vi "Emulate Licor output GV.vi"() -> ()   [LabVIEW 2017, in "Licor-Steuerung.lvlib"]
uses:
  Licor-Steuerung.lvlib
  LicorLI7000/conventions/output line.ctl
  LicorLI7000/LicorLI7000.lvlib
panel:
  in  "Emulator Daten":T1[](array[typedef]) {"time (global)" format="%<%H:%M:%S\n%d/%m/%Y>T"}
  in  "Emulator an?":bool
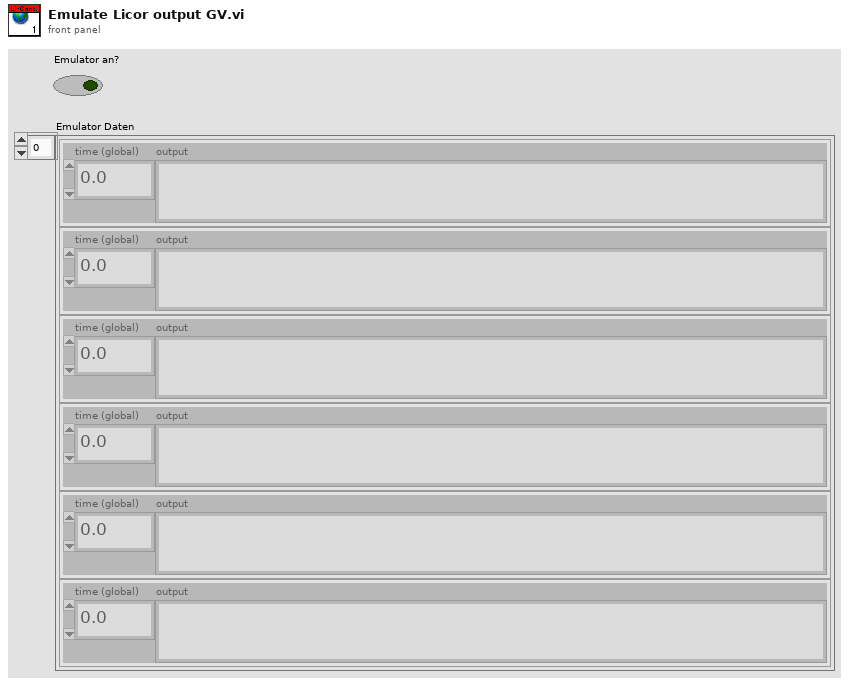
[diagram p1: front panel]
types:
  T1 = typedef "LicorLI7000.lvlib/output line.ctl" = cluster{"time (global)":dbl, "output":string}
diagram:
